vi "test_Basic Write.vi"(8 "error in (no error)":errorcluster, 11 "Scalar Channels Testing in":refnum<class "FPGA Addon Test Class.lvclass">) -> (0 "error out":errorcluster, 3 "Scalar Channels Testing out":refnum<class "FPGA Addon Test Class.lvclass">)   [LabVIEW 2019]
uses:
  FPGA Addon Test Class.lvclass
  C:/Program Files (x86)/National Instruments/LabVIEW 2019/vi.lib/NI/NI VeriStand Development Tools/NI Veristand Test Utilities/VeriStandTestCase/VeriStandTestCase.lvclass
  FPGA Addon Test Class.lvclass/FPGA Addon Test Class.ctl
  <vilib>/NI VeriStand/Execution/Workspace/NI VeriStand - Set Single Channel Value.vi
  <vilib>/NI VeriStand/Execution/Workspace/NI_VS Workspace ExecutionAPI.lvlib
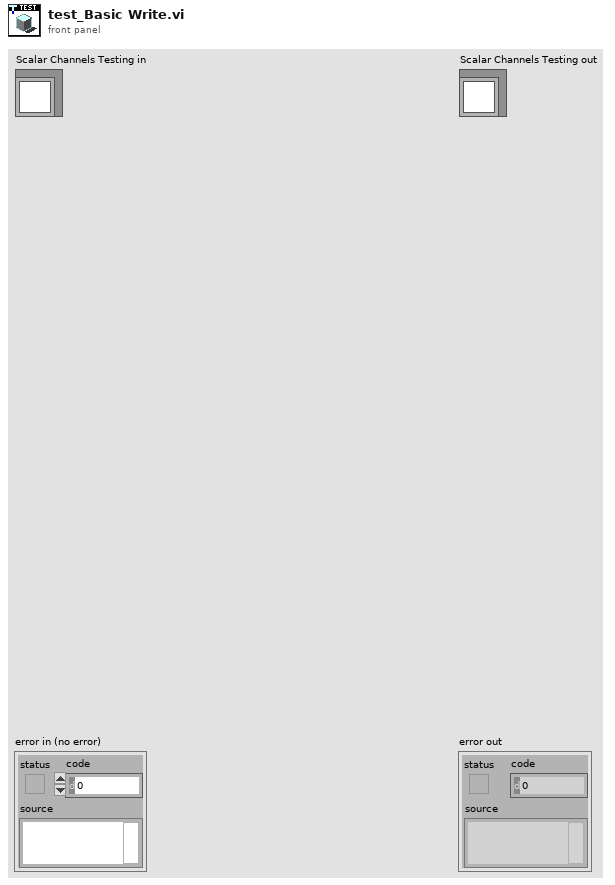
[diagram p1: front panel]
types:
  T1 = typedef "NI_VS Workspace ExecutionAPI.lvlib/WorkspaceAPI.ctl" = refnum<k24>
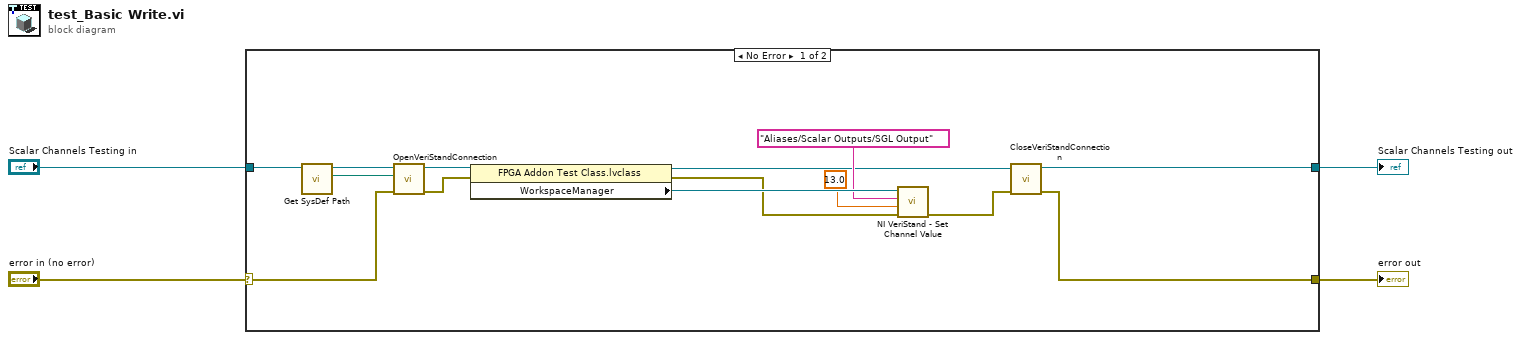
[diagram p0: block diagram]
diagram:
  n1 = case shown="No Error" "error in (no error)" {
    selector: "error in (no error)" -> [w5 w20]
    tunnel: [w17 w20] -> w3
    tunnel: [w18 w19] -> w1
    tunnel: "Scalar Channels Testing in" -> [w8 w19]
    frame No Error {
      n2 = call "Get SysDef Path.vi"("Scalar Channels Testing in"=w8) -> ("SysDef Path"=w6:path, "Scalar Channels Testing out"=w7:refnum<class "FPGA Addon Test Class.lvclass">)  [unwired: 9 in]
      n3 = call-dynamic "OpenVeriStandConnection.vi"("error in (no error)"=w5, "System Definition File"=w6, "VeriStand Test Case in"=w7) -> ("error out"=w15:errorcluster, "VeriStand Test Case out"=w16:refnum<class "FPGA Addon Test Class.lvclass">)  [unwired: 6 in, 1 out]
      n4 = property class="FPGA Addon Test Class.lvclass"(reference=w16, error in=w15) -> (reference out=w10:refnum<class "FPGA Addon Test Class.lvclass">, error out=w11:errorcluster, "WorkspaceManager"=w14:T1)
      n5 = call-poly <vilib>:"NI VeriStand - Set Channel Value.vi"("error in (no error)"=w11, "Value"=13.0, "Channel"="Aliases/Scalar Outputs/SGL Output", "WorkspaceManager in"=w14) -> ("error out"=w9:errorcluster)  [unwired: 6 in, 1 out]
      n6 = call-dynamic "CloseVeriStandConnection.vi"("error in (no error)"=w9, "VeriStand Test Case in"=w10) -> ("error out"=w17:errorcluster, "VeriStand Test Case out"=w18:refnum<class "FPGA Addon Test Class.lvclass">)  [unwired: 8 in]
    }
    frame Error {
    }
  }
  "error out" <- w3
  "Scalar Channels Testing out" <- w1
